vi "nastro.vi"() -> ()   [LabVIEW 2022 SP3]
panel:
  out "pos fc2":dbl
  out "pos fc1":dbl
  out "larghezza slide":u32
  out "posizione slide":i32
  in  "Slide":dbl(slide) scale=0.0..10.0
  out "3 secondi":bool
  in  "stop":bool
  out "fc2":bool
  out "fc1":bool
  out "indietro":bool
  out "in funzione":bool
  in  "start":bool
  out "avanti":bool
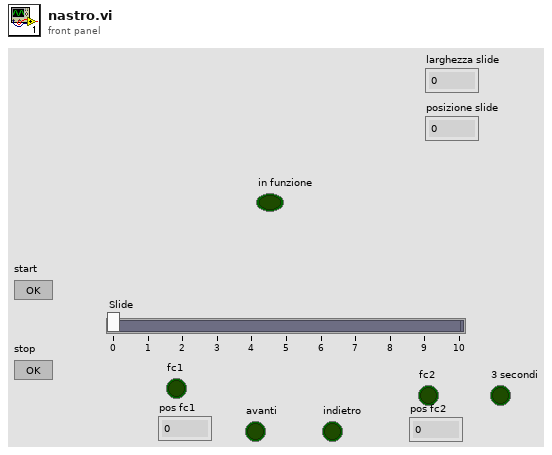
[diagram p1: front panel]
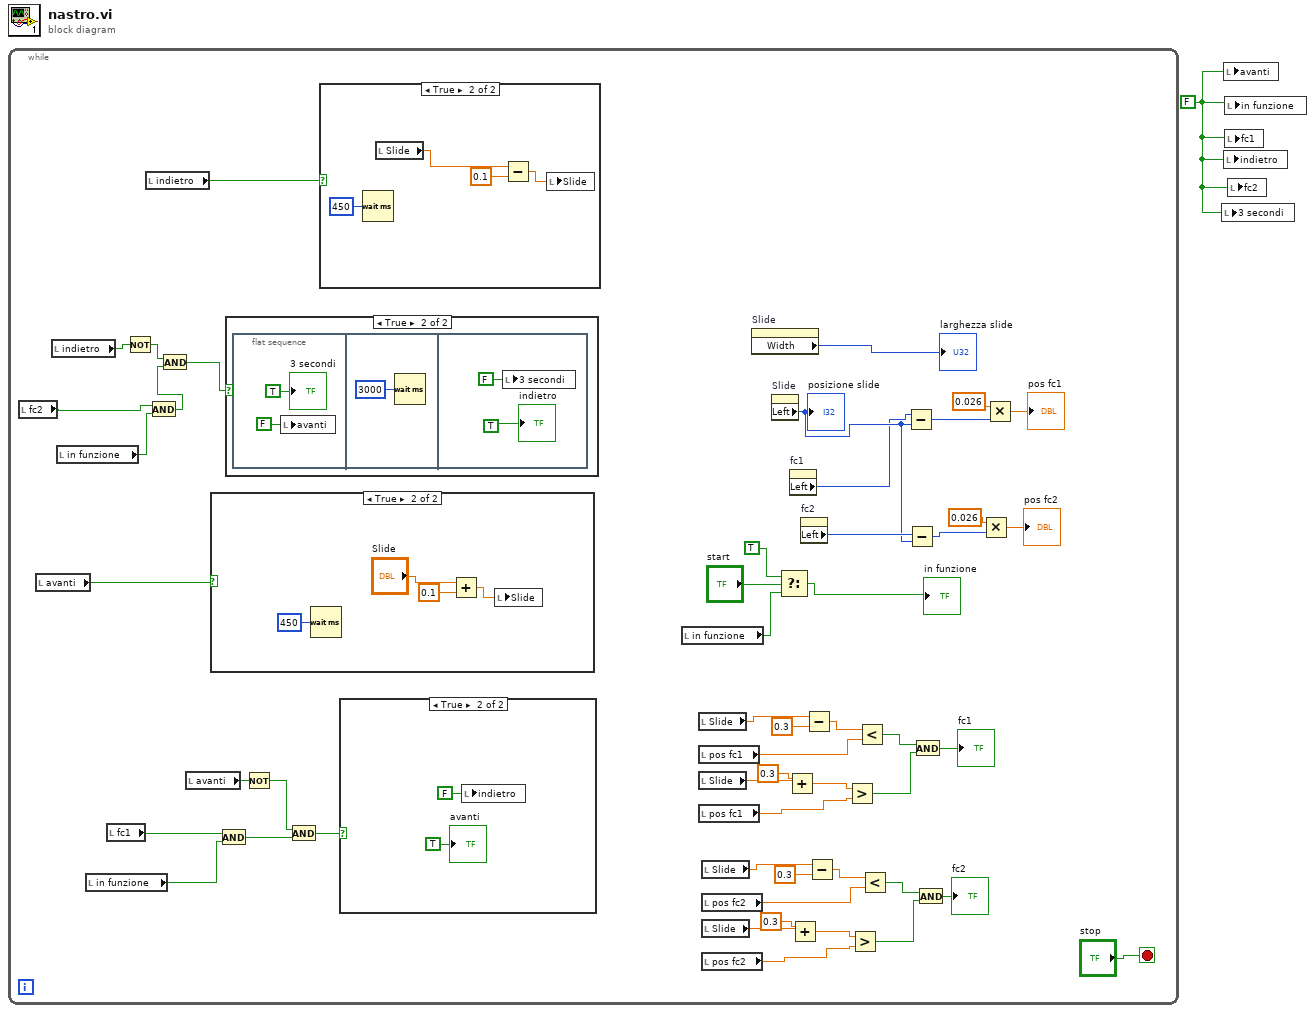
[diagram p0: block diagram]
diagram:
  w1 = FALSE
  n1 = while {
    stop <- "stop" stop-if-true
    n2 = local read "fc2"() -> (w16:bool)
    n3 = local read "avanti"() -> (w43:bool)
    n4 = local read "indietro"() -> (w11:bool)
    n5 = local read "in funzione"() -> (w15:bool)
    n6 = local read "in funzione"() -> (w41:bool)
    n7 = local read "fc1"() -> (w30:bool)
    n8 = Not(x=w11) -> (.not. x?=w12:bool)
    n9 = local read "indietro"() -> (w14:bool)
    n10 = And(x=w16, y=w15) -> (x .and. y?=w13:bool)
    n11 = And(x=w12, y=w13) -> (x .and. y?=w10:bool)
    n12 = local read "avanti"() -> (w7:bool)
    n13 = case shown="True" w43 {
      frame False {
      }
      frame True {
        n14 = Wait (ms)(milliseconds to wait=u32 450) -> ()  [unwired: 1 out]
        n15 = Add(x="Slide", y=0.1) -> (x+y=w60:dbl)
        n16 = local write "Slide"(w60) -> ()
      }
    }
    n17 = And(x=w30, y=w41) -> (x .and. y?=w9:bool)
    n18 = case shown="True" w10 {
      frame False {
      }
      frame True {
        n19 = flat-sequence {
          frame #0 {
            n20 = local write "avanti"(FALSE ("avanti")) -> ()
            "3 secondi" <- TRUE ("3 secondi")
          }
          frame #1 {
            n21 = Wait (ms)(milliseconds to wait=u32 3000) -> ()  [unwired: 1 out]
          }
          frame #2 {
            n22 = local write "3 secondi"(FALSE ("3 secondi")) -> ()
            "indietro" <- TRUE ("indietro")
          }
        }
      }
    }
    n23 = Not(x=w7) -> (.not. x?=w6:bool)
    n24 = And(x=w6, y=w9) -> (x .and. y?=w8:bool)
    n25 = case shown="True" w14 {
      frame False {
      }
      frame True {
        n26 = Wait (ms)(milliseconds to wait=u32 450) -> ()  [unwired: 1 out]
        n27 = local read "Slide"() -> (w53:dbl)
        n28 = Subtract(x=w53, y=0.1) -> (x-y=w55:dbl)
        n29 = local write "Slide"(w55) -> ()
      }
    }
    n30 = case shown="True" w8 {
      frame False {
      }
      frame True {
        n31 = local write "indietro"(FALSE ("indietro")) -> ()
        "avanti" <- TRUE ("avanti")
      }
    }
    n32 = local read "in funzione"() -> (w2:bool)
    n33 = local read "Slide"() -> (w27:dbl)
    n34 = local read "pos fc1"() -> (w21:dbl)
    n35 = local read "Slide"() -> (w23:dbl)
    n36 = local read "pos fc1"() -> (w19:dbl)
    n37 = local read "Slide"() -> (w32:dbl)
    n38 = local read "pos fc2"() -> (w38:dbl)
    n39 = local read "Slide"() -> (w36:dbl)
    n40 = local read "pos fc2"() -> (w40:dbl)
    n41 = property on="Slide" class="Slide (strict)"() -> ("Width"=→"larghezza slide":u32)  [unwired: 2 in, 2 out]
    n42 = property on="Slide" class="Slide (strict)"() -> ("Left"=w47:i32)  [unwired: 2 in, 2 out]
    "posizione slide" <- w47
    n43 = Select(t=TRUE, s="start", f=w2) -> (s? t:f=→"in funzione":bool)
    n44 = Add(x=0.3, y=w23) -> (x+y=w20:dbl)
    n45 = property on="fc1" class="Bool (strict)"() -> ("Left"=w29:i32)  [unwired: 2 in, 2 out]
    n46 = Add(x=0.3, y=w36) -> (x+y=w39:dbl)
    n47 = property on="fc2" class="Bool (strict)"() -> ("Left"=w48:i32)  [unwired: 2 in, 2 out]
    n48 = Subtract(x=w27, y=0.3) -> (x-y=w26:dbl)
    n49 = Subtract(x=w32, y=0.3) -> (x-y=w33:dbl)
    n50 = Greater?(x=w20, y=w19) -> (0:w22:bool)
    n51 = Greater?(x=w39, y=w40) -> (0:w37:bool)
    n52 = Less?(x=w26, y=w21) -> (x < y?=w24:bool)
    n53 = Less?(x=w33, y=w38) -> (x < y?=w35:bool)
    n54 = Subtract(x=w29, y=w47) -> (x-y=w50:i32)
    n55 = Subtract(x=w48, y=w47) -> (x-y=w46:i32)
    n56 = And(x=w24, y=w22) -> (x .and. y?=→"fc1":bool)
    n57 = And(x=w35, y=w37) -> (x .and. y?=→"fc2":bool)
    n58 = Multiply(x=0.026, y=w46) -> (x*y=→"pos fc2":dbl)
    n59 = Multiply(x=0.026, y=w50) -> (x*y=→"pos fc1":dbl)
  }
  n60 = local write "3 secondi"(w1) -> ()
  n61 = local write "avanti"(w1) -> ()
  n62 = local write "indietro"(w1) -> ()
  n63 = local write "in funzione"(w1) -> ()
  n64 = local write "fc1"(w1) -> ()
  n65 = local write "fc2"(w1) -> ()
